vi "Update Descriptions.vi"() -> ()   [LabVIEW 2017]
uses:
  <vilib>/xml/Load XML File.vi
  <vilib>/xml/Close Reference(NNMap).vi
  <vilib>/xml/Close Reference(Node).vi
  <vilib>/xml/NI_XML.lvlib
  <resource>/objmgr/DOMUserDefRef.rc
panel:
  out "error out":errorcluster
  in  "Path":path=path "../Descriptions.xml"
  # "When executed, takes the titles and descriptions from file and applies them\nto the corresponding VI."
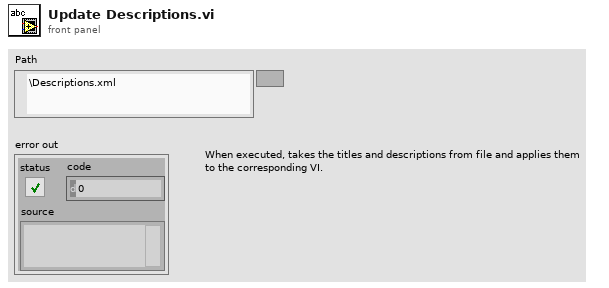
[diagram p1: front panel]
types:
  T1 = cluster{"path":string, "title":string, "description":string}
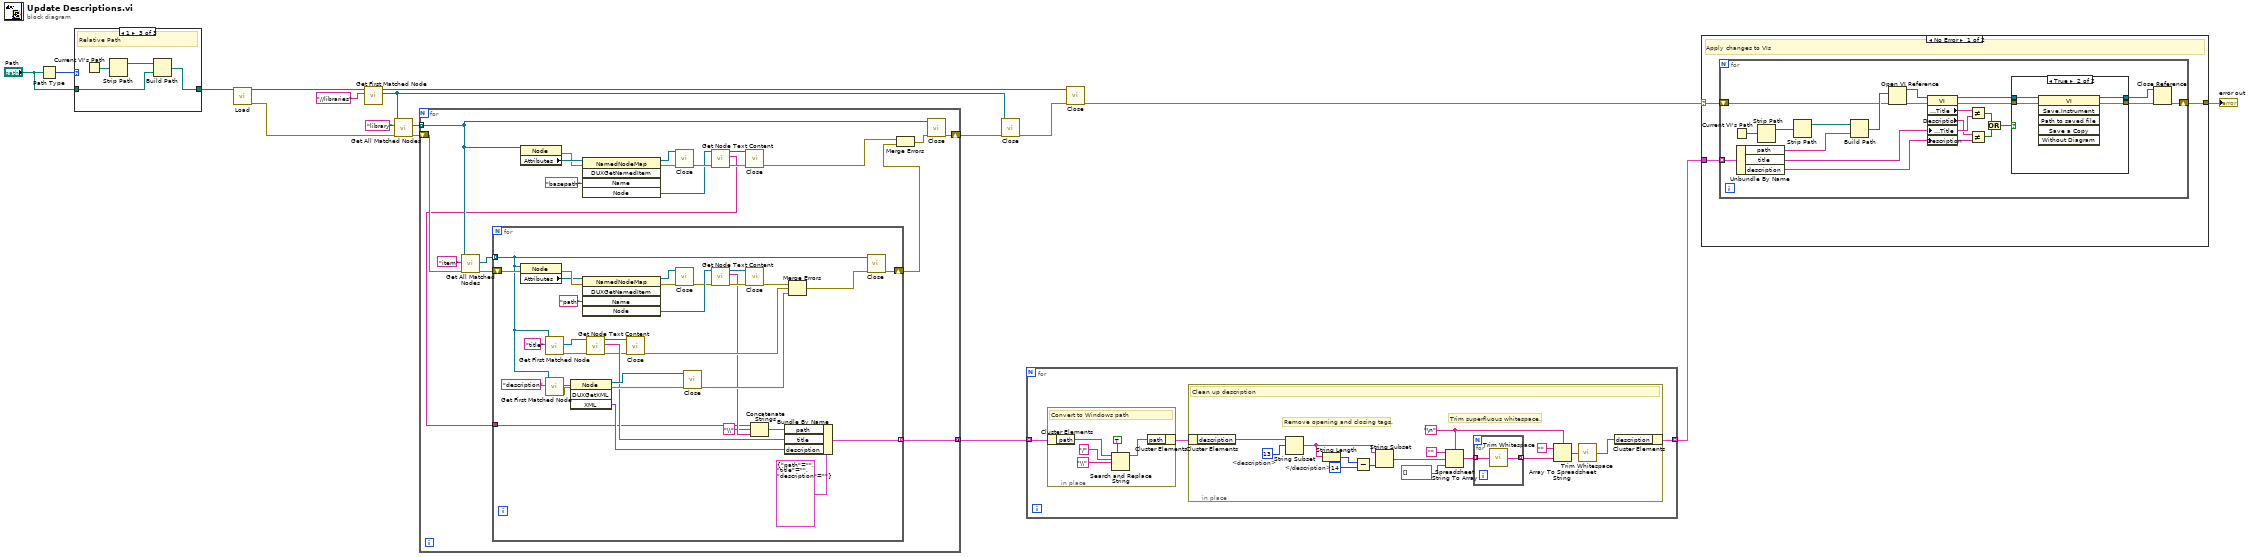
[diagram p0: block diagram]
diagram:
  n1 = Path Type(1:"Path") -> (0:w17:i16)
  n2 = case shown="1" w17 {
    tunnel: "Path" -> [_ w18 w19]
    tunnel: [_ w18 w22] -> w15
    frame Default {
      # "<Not A Path>"
    }
    frame 0 {
      # "Absolute Path"
    }
    frame 1 {
      # "Relative Path"
      n3 = Current VI's Path() -> (path=w21:path)
      n4 = Strip Path(path=w21) -> (stripped path=w20:path)  [unwired: 1 out]
      n5 = Build Path(base path=w20, name or relative path=w19) -> (appended path=w22:path)
    }
  }
  n6 = call-poly <vilib>:"Load.vi"("path to XML document"=w15) -> ("DOM document out"=w5:refnum<k20>, "error out"=w13:errorcluster)  [unwired: 12 in, 1 out]
  n7 = call <vilib>:"Get First Matched Node.vi"("XPath expression"="//libraries", "node in"=w5) -> ("node result"=w1:refnum<k20>, "node out"=w4:refnum<k20>)  [unwired: 7 in, 1 out]
  n8 = call <vilib>:"Get All Matched Nodes.vi"("error in (no error)"=w13, "XPath expression"="library", "node in"=w1) -> ("error out"=w12:errorcluster, "node result array"=w6:refnum<k20>[])  [unwired: 6 in, 1 out]
  n9 = for {
    tunnel: [w37] -> w8 mode=concatenating
    shift-right: [w42] -> w3
    shift-left: w12 -> [w41]
    tunnel: w6 -> [w27] mode=indexing
    n10 = call <vilib>:"Get All Matched Nodes.vi"("error in (no error)"=w41, "XPath expression"="item", "node in"=w27) -> ("error out"=w40:errorcluster, "node result array"=w38:refnum<k20>[])  [unwired: 6 in, 1 out]
    n11 = property class="Node"(reference=w27) -> (error out=w28:errorcluster, "Attributes"=w31:refnum<k20>)  [unwired: 1 in, 1 out]
    n12 = invoke class="NamedNodeMap" method="DUXGetNamedItem"(reference=w31, error in=w28, "Name"="basepath") -> (reference out=w32:refnum<k20>, error out=w30:errorcluster, "Node"=w33:refnum<k20>)  [unwired: 2 in, 2 out]
    n13 = call-poly <vilib>:"Close.vi"("error in (no error)"=w30, "named node map"=w32) -> ("error out"=w34:errorcluster)  [unwired: 7 in]
    n14 = call <vilib>:"Get Node Text Content.vi"("error in (no error)"=w34, "node in"=w33) -> ("error out"=w35:errorcluster, "node text"=w26:string, "node out"=w36:refnum<k20>)  [unwired: 7 in]
    n15 = for {
      tunnel: w38 -> [w63] mode=indexing
      shift-right: [w76] -> w24
      shift-left: w40 -> [w75]
      tunnel: [w68] -> w37 mode=indexing
      tunnel: w26 -> [w43]
      n16 = property class="Node"(reference=w63, error in=w75) -> (error out=w74:errorcluster, "Attributes"=w71:refnum<k20>)  [unwired: 1 out]
      n17 = call <vilib>:"Get First Matched Node.vi"("XPath expression"="title", "node in"=w63) -> ("error out"=w51:errorcluster, "node result"=w61:refnum<k20>)  [unwired: 7 in, 1 out]
      n18 = call <vilib>:"Get First Matched Node.vi"("XPath expression"="description", "node in"=w63) -> ("error out"=w60:errorcluster, "node result"=w59:refnum<k20>)  [unwired: 7 in, 1 out]
      n19 = invoke class="Node" method="DUXGetXML"(reference=w59, error in=w60) -> (reference out=w58:refnum<k20>, error out=w57:errorcluster, "XML"=w48:string)  [unwired: 2 in, 1 out]
      n20 = invoke class="NamedNodeMap" method="DUXGetNamedItem"(reference=w71, error in=w74, "Name"="path") -> (reference out=w70:refnum<k20>, error out=w72:errorcluster, "Node"=w67:refnum<k20>)  [unwired: 2 in, 2 out]
      n21 = call <vilib>:"Get Node Text Content.vi"("error in (no error)"=w51, "node in"=w61) -> ("error out"=w49:errorcluster, "node text"=w50:string, "node out"=w56:refnum<k20>)  [unwired: 7 in]
      n22 = call-poly <vilib>:"Close.vi"("error in (no error)"=w49, "node"=w56) -> ("error out"=w55:errorcluster)  [unwired: 7 in]
      n23 = call-poly <vilib>:"Close.vi"("error in (no error)"=w72, "named node map"=w70) -> ("error out"=w66:errorcluster)  [unwired: 7 in]
      n24 = call-poly <vilib>:"Close.vi"("error in (no error)"=w57, "node"=w58) -> ("error out"=w54:errorcluster)  [unwired: 7 in]
      n25 = call <vilib>:"Get Node Text Content.vi"("error in (no error)"=w66, "node in"=w67) -> ("error out"=w65:errorcluster, "node text"=w46:string, "node out"=w64:refnum<k20>)  [unwired: 7 in]
      n26 = call-poly <vilib>:"Close.vi"("error in (no error)"=w65, "node"=w64) -> ("error out"=w53:errorcluster)  [unwired: 7 in]
      n27 = Concatenate Strings(w43, "\\" ("string"), w46) -> (w45:string)
      n28 = Bundle By Name(cluster=T1 {"path"="", "title"="", "description"=""}, "path"=w45, "title"=w50, "description"=w48) -> (w68:T1)
      n29 = Merge Errors(w53, w55, w54) -> (w52:errorcluster)
      n30 = call-poly <vilib>:"Close.vi"("error in (no error)"=w52, "node"=w63) -> ("error out"=w76:errorcluster)  [unwired: 7 in]
    }
    n31 = call-poly <vilib>:"Close.vi"("error in (no error)"=w35, "node"=w36) -> ("error out"=w25:errorcluster)  [unwired: 7 in]
    n32 = Merge Errors(w25, w24) -> (w23:errorcluster)
    n33 = call-poly <vilib>:"Close.vi"("error in (no error)"=w23, "node"=w27) -> ("error out"=w42:errorcluster)  [unwired: 7 in]
  }
  n34 = call-poly <vilib>:"Close.vi"("error in (no error)"=w3, "node"=w1) -> ("error out"=w2:errorcluster)  [unwired: 7 in]
  n35 = for {
    tunnel: [w77] -> w9 mode=indexing
    tunnel: w8 -> [w79] mode=indexing
    n36 = in-place {
      # "Convert to Windows path"
      n37 = in-place-cluster #1(w79) -> ("path"=w98:string)
      n38 = Search and Replace String(replace all?=TRUE ("replace all? (F)"), input string=w98, search string="/", replace string="\\" ("replace string (\"\")")) -> (result string=w97:string)  [unwired: 4 in, 3 out]
      n39 = in-place-cluster #1("path"=w97) -> (w78:T1)
    }
    n40 = in-place {
      w87 = "\n"
      w84 = 14  # </description>
      w83 = 13  # <description>
      # "Trim superfluous whitespace."
      # "Remove opening and closing tags."
      # "Clean up description"
      n41 = in-place-cluster #2(w78) -> ("description"=w85:string)
      n42 = String Subset(string=w85, offset (0)=w83) -> (substring=w94:string)  [unwired: 1 in]
      n43 = String Length(string=w94) -> (length=w93:i32)
      n44 = Subtract(x=w93, y=w84) -> (x-y=w92:i32)
      n45 = String Subset(string=w94, length (rest)=w92) -> (substring=w91:string)  [unwired: 1 in]
      n46 = Spreadsheet String To Array(delimiter (Tab)=w87, format string="", spreadsheet string=w91, array type (2D Dbl)=string[] []) -> (array=w89:string[])
      n47 = for {
        tunnel: w89 -> [w96] mode=indexing
        tunnel: [w95] -> w88 mode=indexing
        n48 = call <vilib>:"Trim Whitespace.vi"("string"=w96) -> ("trimmed string"=w95:string)  [unwired: 1 in]
      }
      n49 = Array To Spreadsheet String(delimiter (Tab)=w87, array=w88, 3:"") -> (spreadsheet string=w81:string)
      n50 = call <vilib>:"Trim Whitespace.vi"("string"=w81) -> ("trimmed string"=w80:string)  [unwired: 1 in]
      n51 = in-place-cluster #2("description"=w80) -> (w77:T1)
    }
  }
  n52 = call-poly <vilib>:"Close.vi"("error in (no error)"=w2, "node"=w4) -> ("error out"=w11:errorcluster)  [unwired: 7 in]
  n53 = case shown="No Error" w11 {
    selector: w11 -> [w102 w132]
    tunnel: [w103 w132] -> w10
    tunnel: w9 -> [w104 _]
    frame No Error {
      # "Apply changes to VIs"
      n54 = for {
        tunnel: w104 -> [w125] mode=indexing
        shift-right: [w117] -> w103
        shift-left: w102 -> [w116]
        n55 = Current VI's Path() -> (path=w115:path)
        n56 = Unbundle By Name(w125) -> ("path"=w114:string, "title"=w113:string, "description"=w111:string)
        n57 = Strip Path(path=w115) -> (stripped path=w106:path)  [unwired: 1 out]
        n58 = Strip Path(path=w106) -> (stripped path=w105:path)  [unwired: 1 out]
        n59 = Build Path(base path=w105, name or relative path=w114) -> (appended path=w124:path)
        n60 = Open VI Reference(vi path=w124, error in (no error)=w116) -> (vi reference=w123:refnum<vi>, error out=w122:errorcluster)  [unwired: 4 in]
        n61 = property class="VI"(reference=w123, error in=w122, "Front Panel.Title"=w113, "Description"=w111) -> (reference out=w120:refnum<vi>, error out=w121:errorcluster, "Front Panel.Title"=w112:string, "Description"=w110:string)
        n62 = Not Equal?(x=w112, y=w113) -> (x != y?=w109:bool)
        n63 = Not Equal?(x=w110, y=w111) -> (x != y?=w108:bool)
        n64 = Or(x=w109, y=w108) -> (x .or. y?=w107:bool)
        n65 = case shown="True" w107 {
          tunnel: w121 -> [w127 w131]
          tunnel: w120 -> [w126 w130]
          tunnel: [w127 w129] -> w119
          tunnel: [w126 w128] -> w118
          frame False {
          }
          frame True {
            n66 = invoke class="VI" method="Save.Instrument"(reference=w130, error in=w131) -> (reference out=w128:refnum<vi>, error out=w129:errorcluster)  [unwired: 4 in, 4 out]
          }
        }
        n67 = Close Reference(reference=w118, error in (no error)=w119) -> (error out=w117:errorcluster)
      }
    }
    frame Error {
    }
  }
  "error out" <- w10
